vi "Calculate Fixed Point Delta.vi"(1 "WordLength":i8, 2 "IntegerWordLength":i8) -> (0 "delta":dbl)   [LabVIEW 2018]
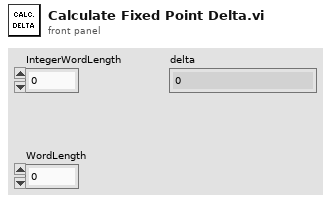
[diagram p1: front panel]
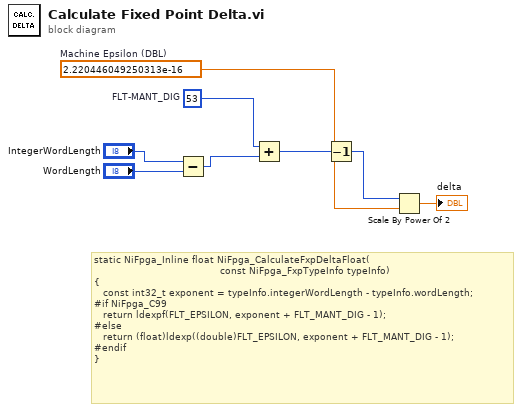
[diagram p0: block diagram]
diagram:
  w5 = i8 53  # FLT-MANT_DIG
  w2 = 2.220446049250313e-16  # Machine Epsilon (DBL)
  # "static NiFpga_Inline float NiFpga_CalculateFxpDeltaFloat(\n                                          const NiFpga_FxpTypeInfo typeInfo)\n{\n   const int32_t exponent = typeInfo.integerWordLength - typeInfo.wordLength;\n#if NiFpga_C99\n   return ldexpf(FLT_EPSILON, exponent + FLT_MANT_DIG - 1);\n#else\n   return (float)ldexp((double)FLT_EPSILON, exponent + FLT_MANT_DIG - 1);\n#endif\n}"
  n1 = Subtract(x="IntegerWordLength", y="WordLength") -> (x-y=w6:i8)
  n2 = Add(x=w5, y=w6) -> (x+y=w4:i8)
  n3 = Decrement(x=w4) -> (x-1=w3:i8)
  n4 = Scale By Power Of 2(n=w3, x=w2) -> (x*2^n=→"delta":dbl)
